vi "Update Feed&Index.vi"(8 "error in (no error)":errorcluster, 11 "Artifactory.VIPM in":refnum<class "Artifactory.VIPM.lvclass">) -> (0 "error out":errorcluster, 2 "Sync'ed Files":path[](array[path]), 3 "Artifactory.VIPM out":refnum<class "Artifactory.VIPM.lvclass">)   [LabVIEW 2021, in "Artifactory.VIPM.lvclass"]
uses:
  Artifactory.VIPM.lvclass
  C:/Repositories/LVOS/Artifactory/lv-src/Artifactory/Artifactory.lvclass
  Artifactory/Artifactory.lvclass/Artifactory.ctl
  Artifactory.VIPM.lvclass/Artifactory.VIPM.ctl
  Artifactory/Artifactory.lvclass
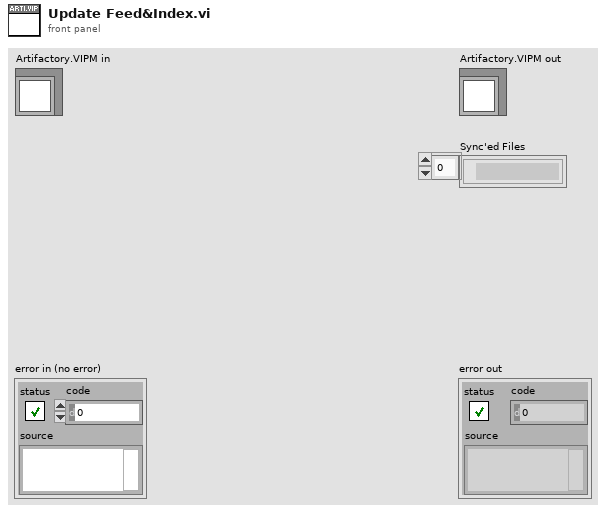
[diagram p1: front panel]
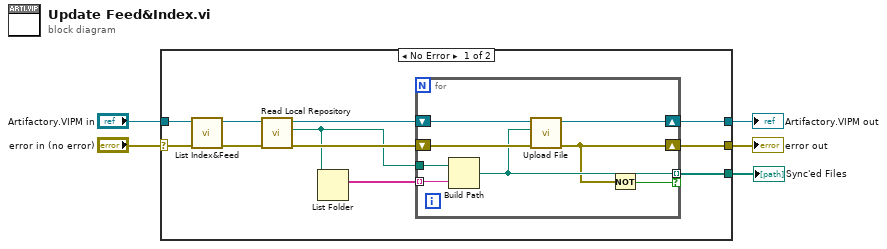
[diagram p0: block diagram]
diagram:
  n1 = case shown="No Error" "error in (no error)" {
    selector: "error in (no error)" -> [w13 w25]
    tunnel: [w12 w25] -> w4
    tunnel: [w15 w24] -> w2
    tunnel: "Artifactory.VIPM in" -> [w14 w24]
    tunnel: [w9 _] -> w1
    frame No Error {
      n2 = call "List Index&Feed.vi"("error in (no error)"=w13, "Artifactory.VIPM in"=w14) -> ("error out"=w8:errorcluster, "Artifactory.VIPM out"=w11:refnum<class "Artifactory.VIPM.lvclass">)  [unwired: 7 in, 1 out]
      n3 = call "Read Local Repository.vi"("Artifactory in"=w11) -> ("Local Repository"=w7:path, "Artifactory out"=w10:refnum<class "Artifactory.VIPM.lvclass">)  [unwired: 9 in]
      n4 = List Folder(path=w7) -> (filenames=w6:string[])  [unwired: 3 in, 3 out]
      n5 = for {
        shift-right: [w22] -> w15
        shift-left: w10 -> [w23]
        shift-right: [w17] -> w12
        shift-left: w8 -> [w21]
        tunnel: w6 -> [w20] mode=indexing
        tunnel: w7 -> [w19]
        tunnel: [w18] -> w9 mode=indexing if=w16
        n6 = Build Path(base path=w19, name or relative path=w20) -> (appended path=w18:path)
        n7 = call "Upload File.vi"("error in (no error)"=w21, "Local File"=w18, "Artifactory in"=w23) -> ("error out"=w17:errorcluster, "Artifactory out"=w22:refnum<class "Artifactory.VIPM.lvclass">)  [unwired: 7 in]
        n8 = Not(x=w17) -> (.not. x?=w16:bool)
      }
    }
    frame Error {
    }
  }
  "error out" <- w4
  "Artifactory.VIPM out" <- w2
  "Sync'ed Files" <- w1
